vi "Update Front Panel Origin.vi"(8 "error in (no error)":errorcluster, 11 "WebFrontPanel in":refnum<class "Web Front Panel.lvclass">) -> (0 "error out":errorcluster, 3 "WebFrontPanel out":refnum<class "Web Front Panel.lvclass">)   [LabVIEW 2015, in "Front Panel Publisher.lvlib" / "Web Front Panel.lvclass"]
uses:
  Web Front Panel.lvclass
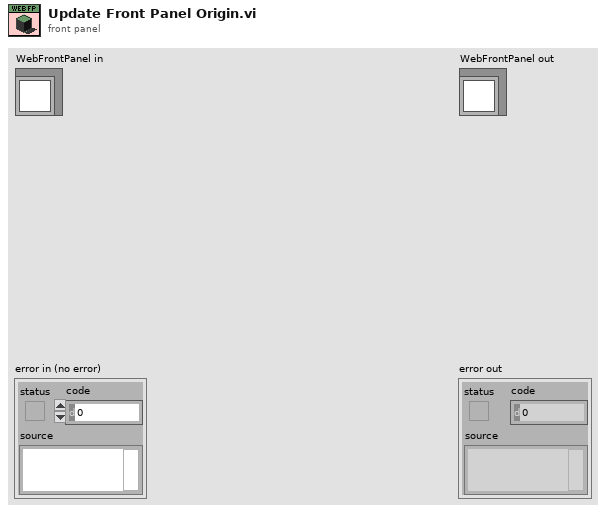
[diagram p1: front panel]
types:
  T1 = typedef "Front Panel Publisher.lvlib/Web Front Panel.lvclass/Object Attributes.ctl" = cluster{"VI Name":string, "VI Reference":refnum<vi>, "Controls":refnum<class "Object.lvclass">[], "Indicators":refnum<class "Object.lvclass">[], "Decorations":refnum<class "Object.lvclass">[], "VR With Previous Get":refnum<data-value>, "VR With Ring Images":refnum<data-value>, "Panel Origin":T2}
  T2 = typedef "LVPointTypeDef.ctl" = cluster{"Horizontal":i16, "Vertical":i16}
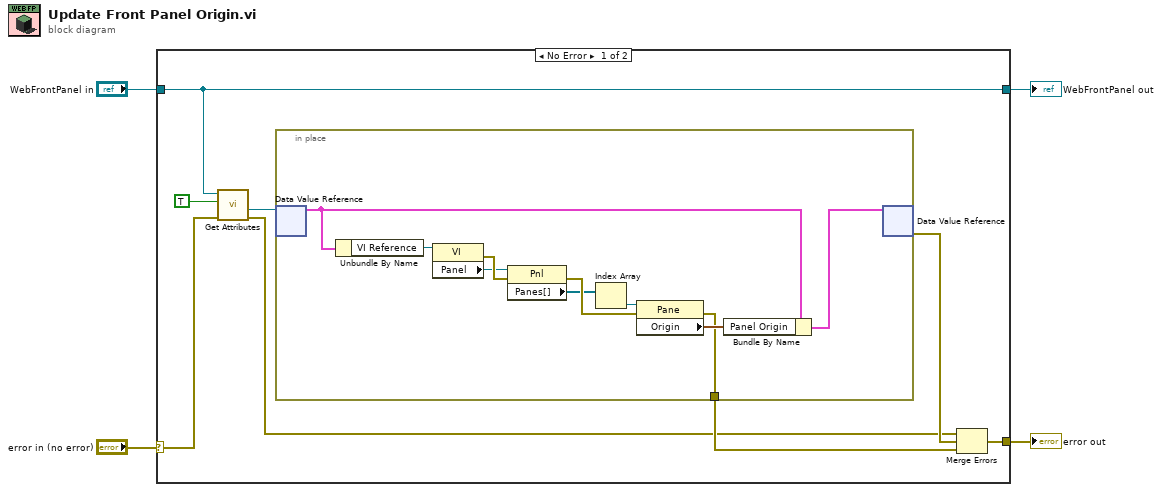
[diagram p0: block diagram]
diagram:
  n1 = case shown="No Error" "error in (no error)" {
    selector: "error in (no error)" -> [w9 w24]
    tunnel: [w5 w24] -> w3
    tunnel: [w11 w23] -> w1
    tunnel: "WebFrontPanel in" -> [w11 w23]
    frame No Error {
      n2 = call "Get Attributes.vi"("error in (no error)"=w9, "Only Get DVR"=TRUE, "Web FP In"=w11) -> ("error out"=w6:errorcluster, "DataRef"=w10:refnum<data-value>)  [unwired: 5 in, 2 out]
      n3 = in-place {
        in-place-border: [w13] -> w7
        n4 = in-place-dvr #1(w10) -> (w21:T1)  [unwired: 1 out]
        n5 = Unbundle By Name(w21) -> ("VI Reference"=w15:refnum<vi>)
        n6 = property class="VI"(reference=w15) -> (error out=w19:errorcluster, "Panel"=w18:refnum<vi>)  [unwired: 1 in, 1 out]
        n7 = property class="Pnl"(reference=w18, error in=w19) -> (error out=w20:errorcluster, "Panes[]"=w17:refnum<vi>[])  [unwired: 1 out]
        n8 = Index Array(array=w17) -> (element=w16:refnum<vi>)  [unwired: 1 in]
        n9 = property class="Pane"(reference=w16, error in=w20) -> (error out=w13:errorcluster, "Origin"=w14:T2)  [unwired: 1 out]
        n10 = Bundle By Name(cluster=w21, "Panel Origin"=w14) -> (w22:T1)
        n11 = in-place-dvr #1(w22) -> (w8:errorcluster)  [unwired: 1 out]
      }
      n12 = Merge Errors(w6, w8, w7) -> (w5:errorcluster)
    }
    frame Error {
    }
  }
  "error out" <- w3
  "WebFrontPanel out" <- w1
